vi "Generate Trap Positiion Waveform.vi"(0 "Base trap positions":dbl[](array[numeric]), 1 "Data Period (s)":dbl, 2 "Input data":dbl[][](array[numeric]), 3 "Position calibration values":dbl[](array[numeric]), 4 "Trap Pos. Disp. Downsample (s)":dbl, 5 "Negate axis":bool[](array[boolean]), 8 "Time Stamp":timestamp) -> (6 "Output waveforms":waveform(dbl)[](array[waveform]))   [LabVIEW 2014]
panel:
  out "Display Period (s)":dbl=0.15 caption="Period (s)" format="%#_6p"
  in  "BD 1 Frequency 1 (MHz)":dbl=70.0 caption="T1 X (MHz)" min=60.0 max=90.0 step=1.0 format="%#_6p"
  in  "BD 1 Frequency 2 (MHz)":dbl=90.0 caption="T2 X (MHz)" min=60.0 max=90.0 step=1.0 format="%#_6p"
  in  "AOM X Cal (nm/MHz)":dbl=169.35
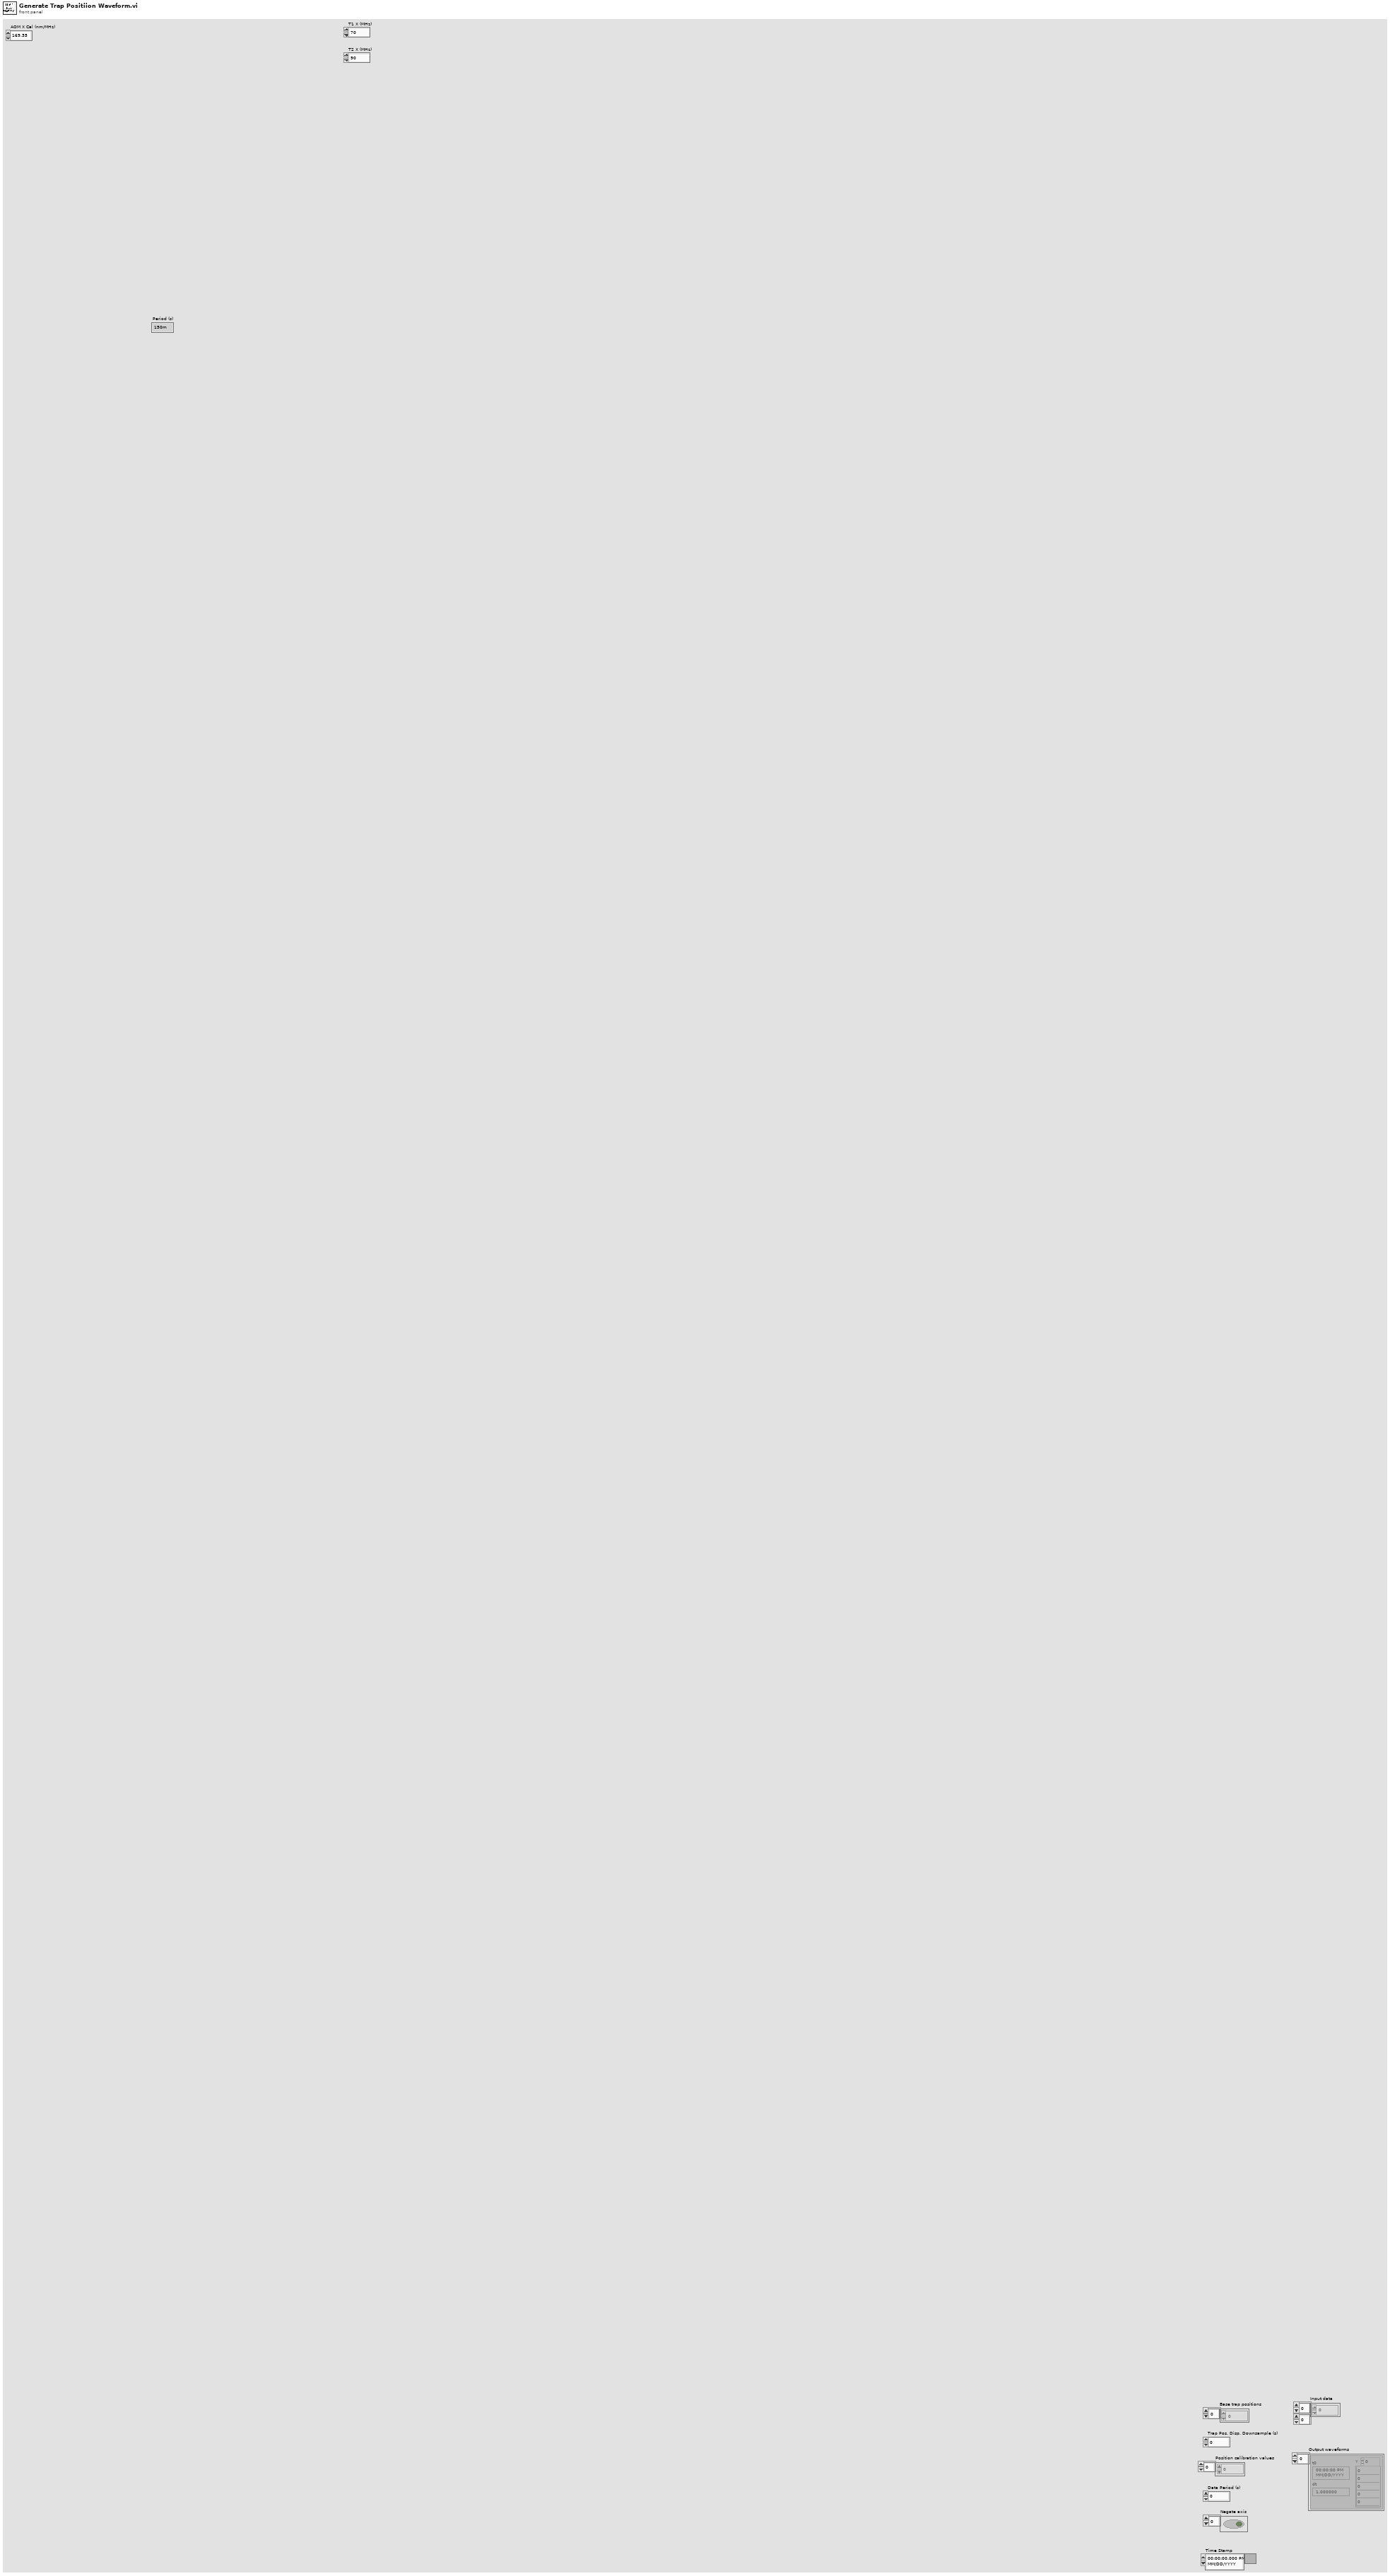
[diagram p1: front panel]
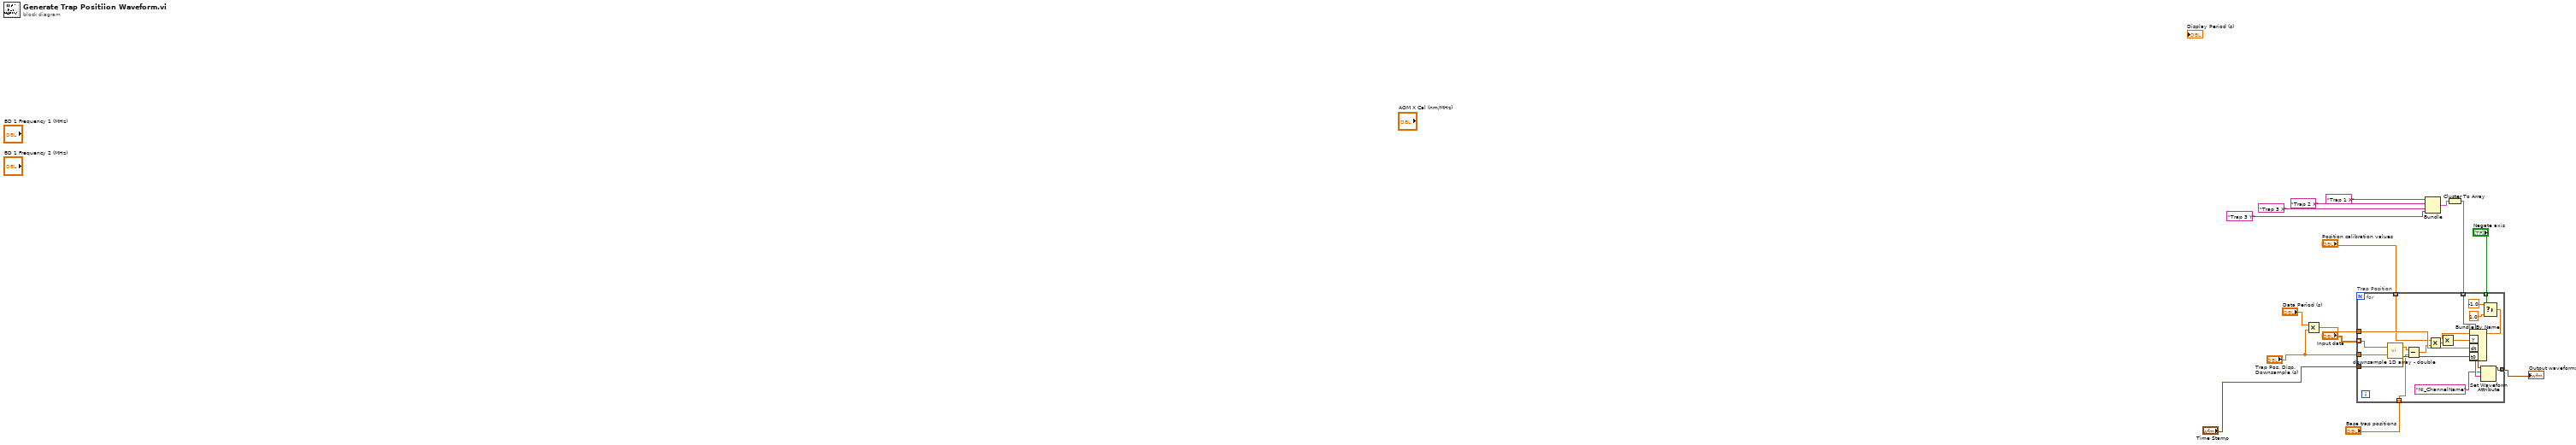
[diagram p0: block diagram]
diagram:
  n1 = Multiply(x="Data Period (s)", y="Trap Pos. Disp. Downsample (s)") -> (x*y=w15:dbl)
  n2 = Bundle("Trap 1 X", "Trap 2 X", "Trap 3 X", "Trap 3 Y") -> (w11:cluster{string, string, string, string})  [unwired: 1 out]
  n3 = Cluster To Array(cluster=w11) -> (array=w14:string[])
  n4 = for "Trap Position" {
    tunnel: "Input data" -> [w33] mode=indexing
    tunnel: "Trap Pos. Disp. Downsample (s)" -> [w32]
    tunnel: w15 -> [w30]
    tunnel: "Time Stamp" -> [w29]
    tunnel: w14 -> [w27] mode=indexing
    tunnel: [w26] -> w2 mode=indexing
    tunnel: "Base trap positions" -> [w24] mode=indexing
    tunnel: "Position calibration values" -> [w22] mode=indexing
    tunnel: "Negate axis" -> [w16] mode=indexing
    n5 = call "downsample 1D array - double.vi"("Ave N"=w32, "Array In"=w33) -> ("Array Out"=w31:dbl[])  [unwired: 1 out]
    n6 = Subtract(x=w31, y=w24) -> (x-y=w25:dbl[])
    n7 = Multiply(x=w22, y=w25) -> (x*y=w23:dbl[])
    n8 = Select(t=-1.0, s=w16, f=1.0) -> (s? t:f=w17:dbl)
    n9 = Multiply(x=w17, y=w23) -> (x*y=w21:dbl[])
    n10 = Bundle By Name("Y"=w21, "dt"=w30, "t0"=w29) -> (w28:waveform(dbl))  [unwired: 1 out]
    n11 = Set Waveform Attribute(5:w27, 6:"NI_ChannelName" ("name"), 7:w28) -> (3:w26:waveform(dbl))  [unwired: 1 in, 2 out]
  }
  "Output waveforms" <- w2
